vi "接收通信报文.vi"(8 "error in (no error)":errorcluster, 11 "串口通信类 in":refnum<class "串口通信类.lvclass">) -> (0 "error out":errorcluster, 1 "接收数据有效？":bool, 2 "接受到的原始报文数据":string, 3 "串口通信类 out":refnum<class "串口通信类.lvclass">)   [LabVIEW 2015, in "串口通信类.lvclass"]
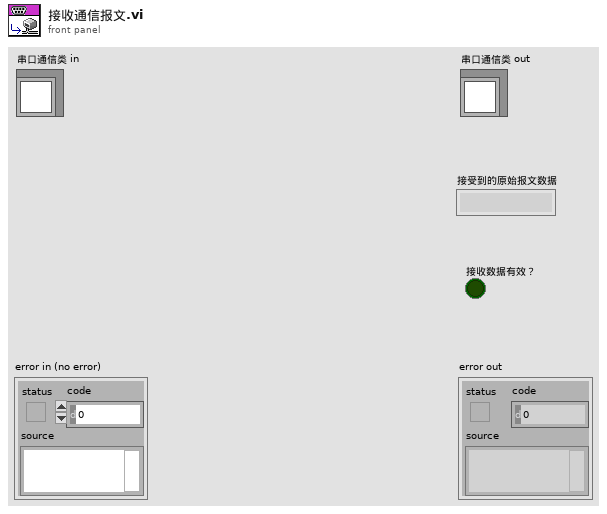
[diagram p1: front panel]
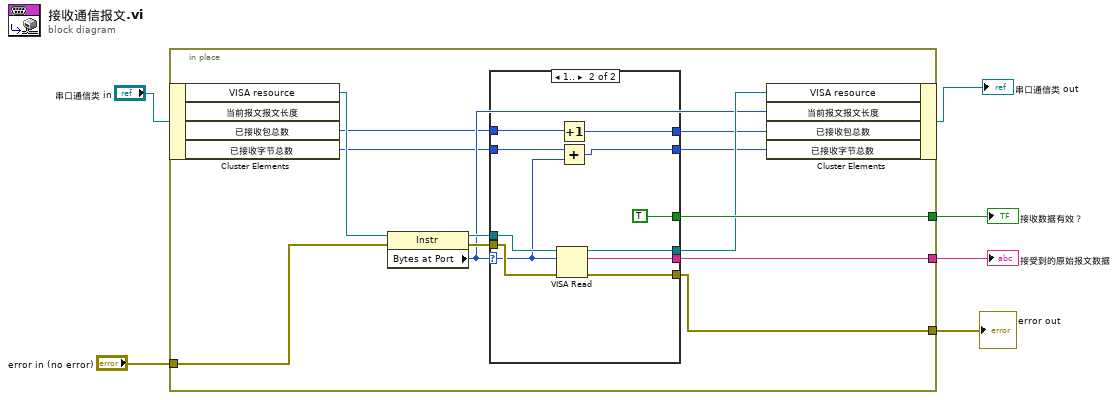
[diagram p0: block diagram]
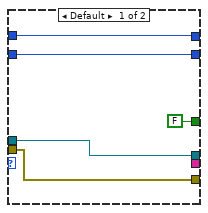
[diagram p2: hidden frame]
diagram:
  n1 = in-place {
    in-place-border: "error in (no error)" -> [w18]
    in-place-border: [w16] -> w5
    in-place-border: [w15] -> w4
    in-place-border: [w7] -> w1
    n2 = in-place-cluster #1("串口通信类 in") -> ("VISA resource"=w14:refnum<visa-resource-name>, "已接收包总数"=w11:u64, "已接收字节总数"=w9:u64)  [unwired: 1 out]
    n3 = property class="Instr"(reference=w14, error in=w18) -> (reference out=w19:refnum<visa-resource-name>, error out=w17:errorcluster, "Bytes at Port"=w12:u32)
    n4 = case shown="1.." w12 {
      selector: w12 -> [_ w26]
      tunnel: w19 -> [w23 w35]
      tunnel: w17 -> [w22 w34]
      tunnel: [_ w33] -> w16
      tunnel: [FALSE TRUE] -> w15
      tunnel: [w23 w31] -> w13
      tunnel: [w22 w30] -> w7
      tunnel: w11 -> [w21 w29]
      tunnel: [w21 w28] -> w10
      tunnel: w9 -> [w20 w27]
      tunnel: [w20 w25] -> w8
      frame Default {
      }
      frame 1.. {
        n5 = VISA Read(VISA resource name=w35, byte count=w26, error in (no error)=w34) -> (VISA resource name out=w31:refnum<visa-resource-name>, read buffer=w33:string, error out=w30:errorcluster)  [unwired: 1 out]
        n6 = Increment(x=w29) -> (x+1=w28:u64)
        n7 = Add(x=w27, y=w26) -> (x+y=w25:u64)
      }
    }
    n8 = in-place-cluster #1("VISA resource"=w13, "当前报文报文长度"=w12, "已接收包总数"=w10, "已接收字节总数"=w8) -> (→"串口通信类 out":refnum<class "串口通信类.lvclass">)
  }
  "error out" <- w1
  "接收数据有效？" <- w4
  "接受到的原始报文数据" <- w5
